vi "Send Script Trigger.vi"(7 "trigger id (script trigger 0)":T1="ScriptTrigger0", 8 "error in (no error)":errorcluster, 10 "Delay Time (s)":dbl=0.001, 11 "HSDIO Sessions In":refnum<k15>[](array[refnum])) -> (0 "error out":errorcluster, 3 "HSDIO Sessions Out":refnum<k15>[](array[refnum]))   [LabVIEW 2013]
doc: "Sends the selected script trigger for HSDIO sessions"
uses:
  <instrlib>/niHSDIO/niHSDIO.llb/niHSDIO_ctl Trigger Script - trigID Values (Ring).ctl
  <instrlib>/niHSDIO/niHSDIO.llb/niHSDIO_ctl Trigger SW - TrigName Values (Ring).ctl
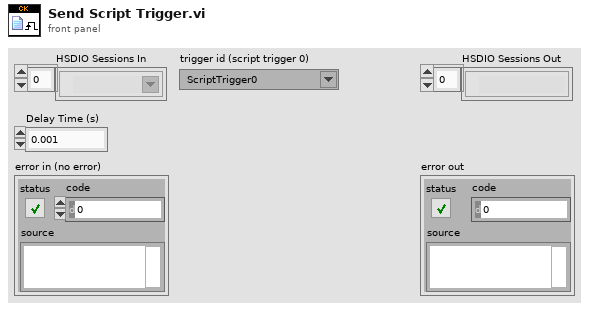
[diagram p1: front panel]
types:
  T1 = typedef "niHSDIO_ctl Trigger Script - trigID Values (Ring).ctl" = string
  T2 = typedef "niHSDIO_ctl Trigger SW - TrigName Values (Ring).ctl" = i32
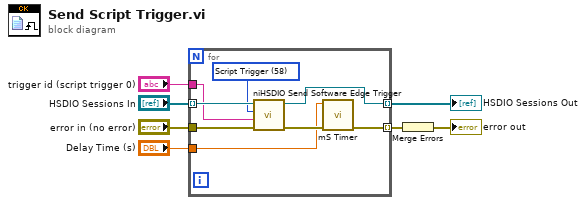
[diagram p0: block diagram]
diagram:
  n1 = for {
    tunnel: "HSDIO Sessions In" -> [w14] mode=indexing
    tunnel: "error in (no error)" -> [w15]
    tunnel: "trigger id (script trigger 0)" -> [w12]
    tunnel: [w9] -> w3 mode=indexing
    tunnel: [w11] -> w2 mode=indexing
    tunnel: "Delay Time (s)" -> [w8]
    w13 = T2 58 items=["Start Trigger"=53, "Reference Trigger"=54, "Advance Trigger"=61, "Script Trigger"=58, "Stop Trigger"=82] ("trigger (start trigger)")
    n2 = call <instrlib>:"niHSDIO Send Software Edge Trigger.vi"("error in (no error)"=w15, "trigger identifier (none)"=w12, "trigger (start trigger)"=w13, "instrument handle"=w14) -> ("error out"=w10:errorcluster, "instrument handle out"=w11:refnum<k15>)  [unwired: 6 in]
    n3 = call "mS Timer.vi"("Error In"=w10, "Delay(S)"=w8) -> ("Error Out"=w9:errorcluster)  [unwired: 9 in]
  }
  "HSDIO Sessions Out" <- w2
  n4 = Merge Errors(w3) -> (→"error out":errorcluster)
